vi "camToPipette_rel_3d.vi"(7 "which manipulator":T2(ring), 9 "transform cluster + actuator":T1, 11 "rel cam (px)":dbl[](array[numeric])) -> (3 "rel pipette (steps)":dbl[](array[numeric]))   [LabVIEW 2015]
uses:
  pipette cleaning/pressure box/cleaning_soft/controls/actuator_type.ctl
  pipette cleaning/pressure box/cleaning_soft/controls/actuator_cluster.ctl
  transform_properties_actuators.ctl
  controls/transform_cluster_actuator.ctl
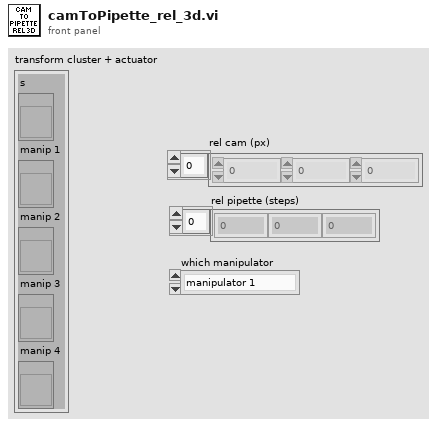
[diagram p1: front panel]
types:
  T1 = typedef "transform_cluster_actuator.ctl" = cluster{"s":refnum<vi>, "manip 1":refnum<vi>, "manip 2":refnum<vi>, "manip 3":refnum<vi>, "manip 4":refnum<vi>}
  T2 = enum16{"manipulator 1", "manipulator 2", "manipulator 3", "manipulator 4"}
  T3 = typedef "transform_properties_actuators.ctl" = cluster{"theta (deg)":dbl, "X sc factor (px/step)":dbl, "Y sc factor (px/step)":dbl, "zero loc (x,y,z)":dbl[], "flip y?":bool, "flip x?":bool, "gamma (deg)":dbl, "flip z?":bool, "Z sc factor (px/step)":dbl, "actuator":T4, "safe space (steps)":i32[]}
  T4 = typedef "actuator_cluster.ctl" = cluster{"Actuator COM":refnum<visa-resource-name>, "Actuator type":T5}
  T5 = typedef "actuator_type.ctl" = enum16{"Scientifica", "Sutter", "Demo", "Off"}
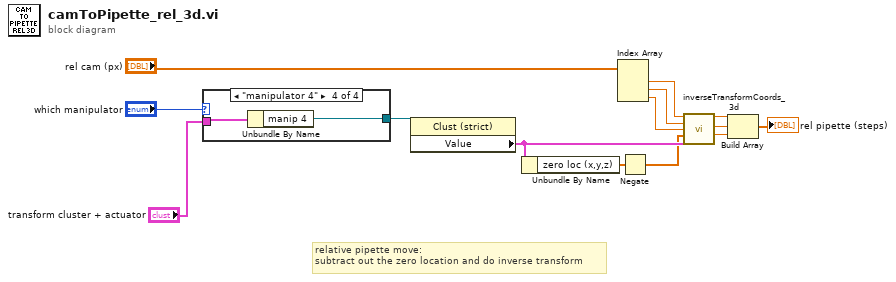
[diagram p0: block diagram]
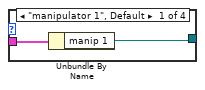
[diagram p2: hidden frame]
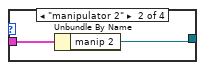
[diagram p3: hidden frame]
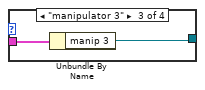
[diagram p4: hidden frame]
diagram:
  # "relative pipette move:\nsubtract out the zero location and do inverse transform"
  n1 = case shown="\"manipulator 4\"" "which manipulator" {
    tunnel: "transform cluster + actuator" -> [w16 w18 w20 w22]
    tunnel: [w15 w17 w19 w21] -> w13
    frame "manipulator 1", Default {
      n2 = Unbundle By Name(w16) -> ("manip 1"=w15:refnum<vi>)
    }
    frame "manipulator 2" {
      n3 = Unbundle By Name(w18) -> ("manip 2"=w17:refnum<vi>)
    }
    frame "manipulator 3" {
      n4 = Unbundle By Name(w20) -> ("manip 3"=w19:refnum<vi>)
    }
    frame "manipulator 4" {
      n5 = Unbundle By Name(w22) -> ("manip 4"=w21:refnum<vi>)
    }
  }
  n6 = property class="Clust (strict)"(reference=w13) -> ("Value"=w6:T3)  [unwired: 1 in, 2 out]
  n7 = Unbundle By Name(w6) -> ("zero loc (x,y,z)"=w5:dbl[])
  n8 = Index Array(array="rel cam (px)") -> (element #1=w11:dbl, element #2=w10:dbl, element #3=w2:dbl)  [unwired: 3 in]
  n9 = Negate(x=w5) -> (-x=w4:dbl[])
  n10 = call "inverseTransformCoords_3d.vi"("x"=w11, "y"=w10, "z"=w2, "current stage pos (px)"=w4, "transform properties"=w6) -> ("x out"=w9:dbl, "y out"=w8:dbl, "z out"=w1:dbl)  [unwired: 8 in]
  n11 = Build Array(w9, w8, w1) -> (→"rel pipette (steps)":dbl[])
